vi "poly_data_queue_double.vi"(6 "initial queue element (NaN)":dbl=nan, 7 "initialize":bool, 8 "Error in":errorcluster caption="Error in (no error)", 10 "sample length":i32=100, 11 "input data point":dbl format="%0.2f") -> (0 "Error out":errorcluster, 2 "Queue":dbl[](array[numeric]), 3 "eliminated element":dbl format="%0.2f", 4 "current length":i32)   [LabVIEW 2015, in "_average_tools_polys.lvlib"]
uses:
  _average_tools_polys.lvlib
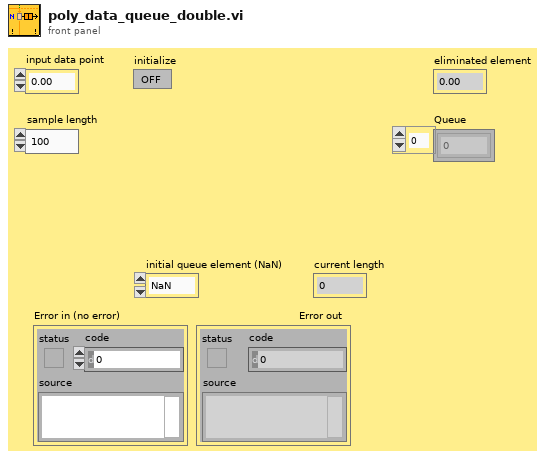
[diagram p1: front panel]
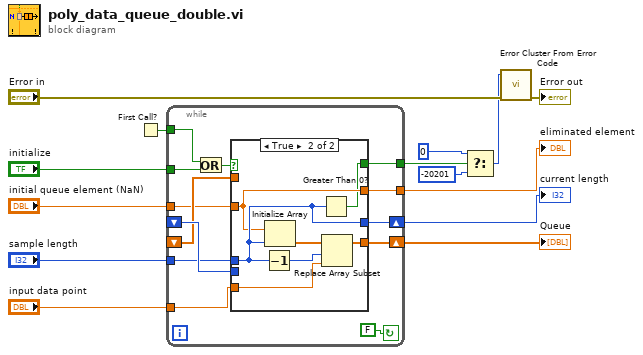
[diagram p0: block diagram]
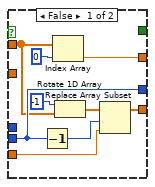
[diagram p2: hidden frame]
diagram:
  n1 = First Call?() -> (First Call?: T/F=w12:bool)
  n2 = while {
    tunnel: w12 -> [w22]
    shift-left: _ -> [w25]
    shift-right: [w26] -> w13
    shift-left: _ -> [w24]
    shift-right: [w27] -> w14
    tunnel: "initialize" -> [w20]
    tunnel: "input data point" -> [w19]
    tunnel: "initial queue element (NaN)" -> [w18]
    tunnel: "sample length" -> [w17]
    tunnel: [w16] -> w7
    tunnel: [w15] -> w2
    stop <- FALSE continue-if-true
    n3 = Or(x=w22, y=w20) -> (x .or. y?=w21:bool)
    n4 = case shown="True" w21 {
      tunnel: [w33 w39] -> w27
      tunnel: [w34 w42] -> w26
      tunnel: w25 -> [w34 _]
      tunnel: w24 -> [w30 _]
      tunnel: w19 -> [w35 w40]
      tunnel: w18 -> [_ w38]
      tunnel: w17 -> [_ w42]
      tunnel: [w28 w38] -> w16
      tunnel: [_ w37] -> w15
      frame False {
        n5 = Decrement(x=w34) -> (x-1=w32:i32)
        n6 = Index Array(array=w30, index=0 ("Index")) -> (element=w28:dbl)
        n7 = Rotate 1D Array(1:w30, 2:i16 -1 ("n")) -> (0:w31:dbl[])
        n8 = Replace Array Subset(array=w31, new element=w35, index=w32) -> (w33:dbl[])
      }
      frame True {
        n9 = Decrement(x=w42) -> (x-1=w43:i32)
        n10 = Initialize Array(w38, w42) -> (w41:dbl[])
        n11 = Greater Than 0?(x=w42) -> (x > 0?=w37:bool)
        n12 = Replace Array Subset(array=w41, new element=w40, index=w43) -> (w39:dbl[])
      }
    }
  }
  "Queue" <- w14
  "current length" <- w13
  "eliminated element" <- w7
  n13 = Select(t=0, s=w2, f=-20201) -> (s? t:f=w1:i32)
  n14 = call <vilib>:"Error Cluster From Error Code.vi"("error in (no error)"="Error in", "error code (0)"=w1) -> ("error out"=→"Error out":errorcluster)  [unwired: 7 in]
